vi "hp_indicator.vi"(10 "HP":i32) -> (2 "HP pic":T1)   [LabVIEW 2025]
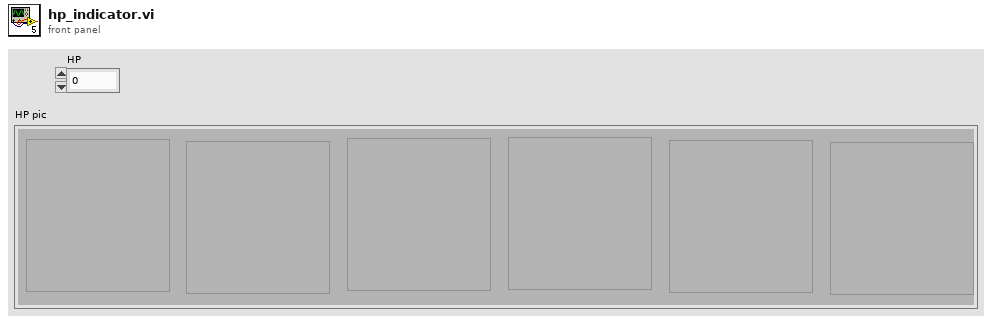
[diagram p1: front panel]
types:
  T1 = cluster{"Boolean":bool, "Boolean 2":bool, "Boolean 3":bool, "Boolean 4":bool, "Boolean 5":bool, "Boolean 6":bool}
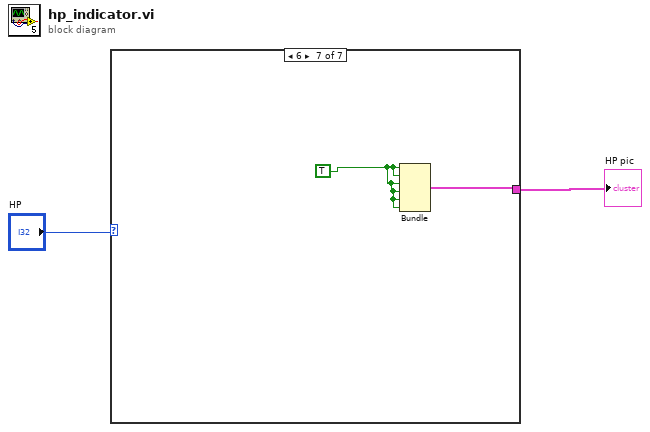
[diagram p0: block diagram]
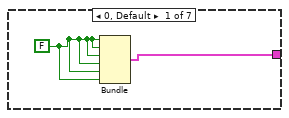
[diagram p2: hidden frame]
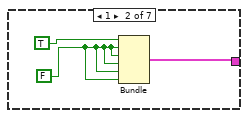
[diagram p3: hidden frame]
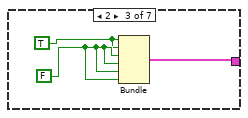
[diagram p4: hidden frame]
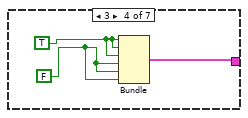
[diagram p5: hidden frame]
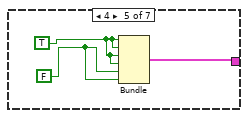
[diagram p6: hidden frame]
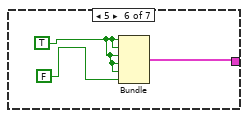
[diagram p7: hidden frame]
diagram:
  n1 = case shown="6" "HP" {
    tunnel: [w3 w5 w9 w13 w16 w19 w21] -> w1
    frame 0, Default {
      w4 = FALSE
      n2 = Bundle(w4, w4, w4, w4, w4, w4) -> (w3:cluster{bool, bool, bool, bool, bool, bool})  [unwired: 1 in]
    }
    frame 1 {
      w6 = FALSE
      n3 = Bundle(TRUE, w6, w6, w6, w6, w6) -> (w5:cluster{bool, bool, bool, bool, bool, bool})  [unwired: 1 in]
    }
    frame 2 {
      w10 = FALSE
      w8 = TRUE
      n4 = Bundle(w8, w8, w10, w10, w10, w10) -> (w9:cluster{bool, bool, bool, bool, bool, bool})  [unwired: 1 in]
    }
    frame 3 {
      w11 = FALSE
      w12 = TRUE
      n5 = Bundle(w12, w12, w12, w11, w11, w11) -> (w13:cluster{bool, bool, bool, bool, bool, bool})  [unwired: 1 in]
    }
    frame 4 {
      w15 = FALSE
      w14 = TRUE
      n6 = Bundle(w14, w14, w14, w14, w15, w15) -> (w16:cluster{bool, bool, bool, bool, bool, bool})  [unwired: 1 in]
    }
    frame 5 {
      w17 = TRUE
      n7 = Bundle(w17, w17, w17, w17, w17, FALSE) -> (w19:cluster{bool, bool, bool, bool, bool, bool})  [unwired: 1 in]
    }
    frame 6 {
      w20 = TRUE
      n8 = Bundle(w20, w20, w20, w20, w20, w20) -> (w21:cluster{bool, bool, bool, bool, bool, bool})  [unwired: 1 in]
    }
  }
  "HP pic" <- w1
